vi "Circle Points.vi"(6 "Phi":dbl, 7 "N":i32=100, 9 "Radius":dbl, 10 "Y":dbl, 11 "X":dbl) -> (2 "Ys":dbl[](array[numeric]), 3 "Xs":dbl[](array[numeric]))   [LabVIEW 2023]
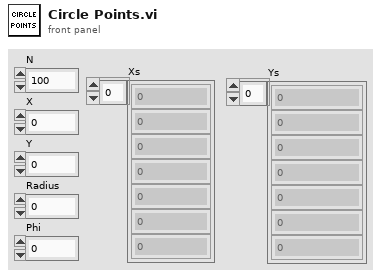
[diagram p1: front panel]
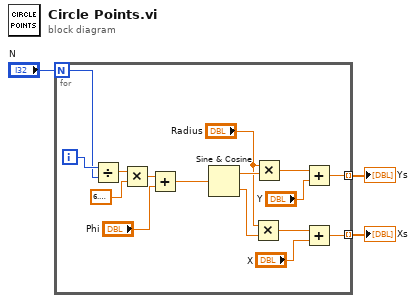
[diagram p0: block diagram]
diagram:
  n1 = for {
    N: "N" -> [w18]
    tunnel: [w5] -> w2 mode=indexing
    tunnel: [w4] -> w1 mode=indexing
    i -> [w19]
    n2 = Divide(x=w19, y=w18) -> (x/y=w17:dbl)
    n3 = Multiply(x=w17, y=6.283185307179586) -> (x*y=w8:dbl)
    n4 = Add(x=w8, y="Phi") -> (x+y=w6:dbl)
    n5 = Sine & Cosine(0:w6) -> (1:w15:dbl, 2:w14:dbl)
    n6 = Multiply(x="Radius", y=w14) -> (x*y=w12:dbl)
    n7 = Multiply(x="Radius", y=w15) -> (x*y=w13:dbl)
    n8 = Add(x=w13, y="Y") -> (x+y=w5:dbl)
    n9 = Add(x=w12, y="X") -> (x+y=w4:dbl)
  }
  "Ys" <- w2
  "Xs" <- w1
